vi "DepthSearch.vi"(6 "Path in":refnum<data-value>[](array[refnum]), 8 "error in (no error)":errorcluster, 10 "GraphNode in":refnum<data-value>, 11 "GraphSearch in":refnum<class "GraphSearch.lvclass">) -> (0 "error out":errorcluster, 1 "found":bool, 2 "GraphNode out":refnum<data-value>, 3 "GraphSearch out":refnum<class "GraphSearch.lvclass">, 4 "Path out":refnum<data-value>[](array[refnum]))   [LabVIEW 2009, in "GraphSearch.lvclass"]
uses:
  GraphSearch.lvclass
  GraphNode/GraphNode.lvclass
  Node/Node.lvclass
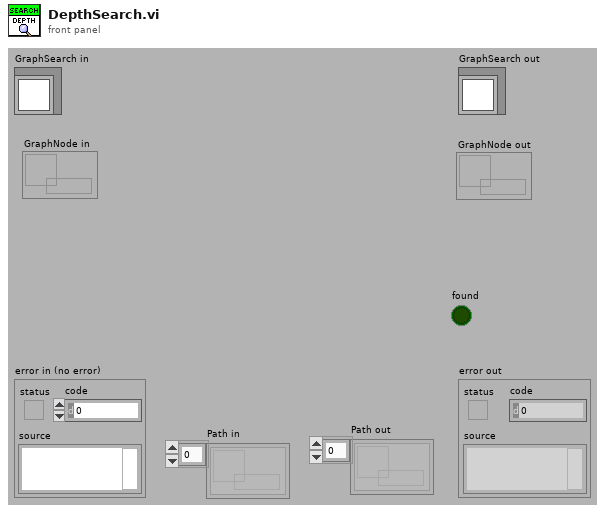
[diagram p1: front panel]
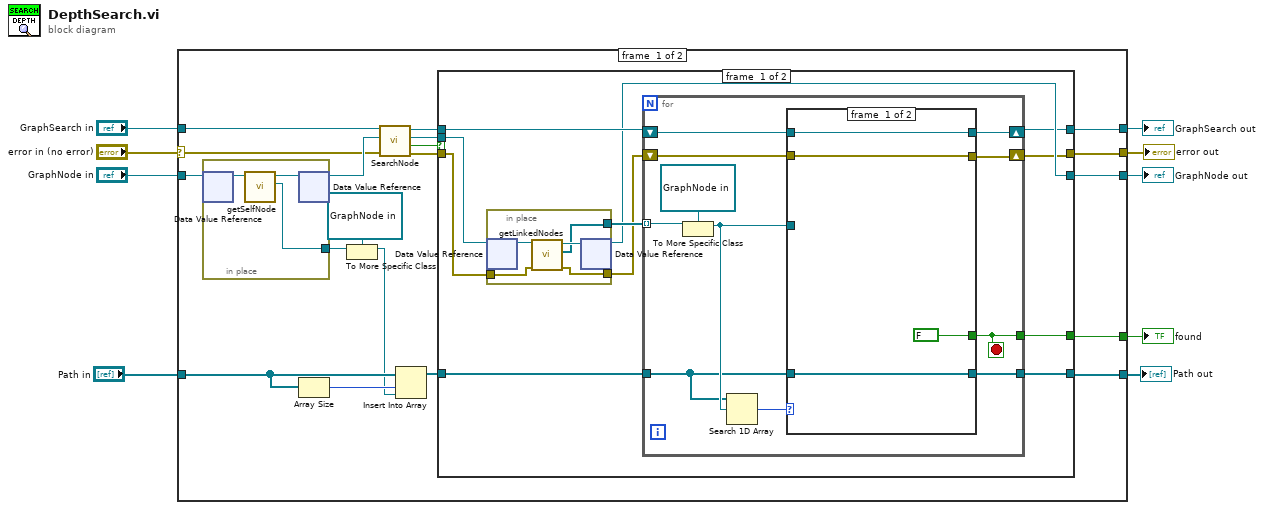
[diagram p0: block diagram]
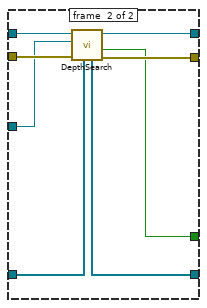
[diagram p2: hidden frame]
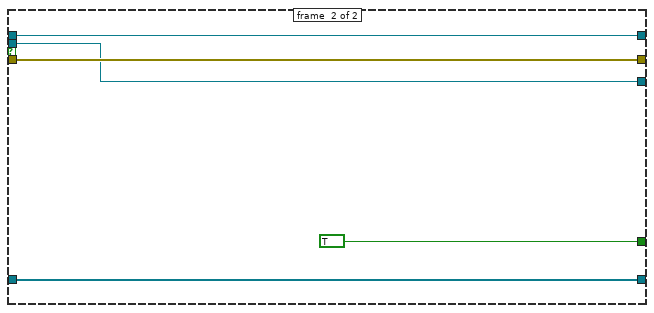
[diagram p3: hidden frame]
diagram:
  n1 = case shown="No Error" "error in (no error)" {
    selector: "error in (no error)" -> [w15 w79]
    tunnel: [w22 w79] -> w8
    tunnel: [w21 w78] -> w6
    tunnel: "GraphSearch in" -> [w19 w78]
    tunnel: "GraphNode in" -> [w18 w77]
    tunnel: "Path in" -> [w13 w76]
    tunnel: [w24 w76] -> w3
    tunnel: [w23 _] -> w2
    tunnel: [w20 w77] -> w1
    frame #0 {
      n2 = in-place {
        in-place-border: [w29] -> w16
        n3 = in-place-dvr #1(w18) -> (w31:refnum<class "GraphNode.lvclass">)  [unwired: 1 out]
        n4 = call "getSelfNode.vi"("Node in"=w31) -> ("selfNode"=w29:refnum<data-value>, "Node out"=w30:refnum<class "GraphNode.lvclass">)  [unwired: 8 in, 1 out]
        n5 = in-place-dvr #1(w30) -> (w17:refnum<data-value>)  [unwired: 1 out]
      }
      n6 = Array Size(array=w13) -> (size(s)=w11:i32)
      n7 = To More Specific Class(target class=refnum<data-value> refnum ("GraphNode out"), reference=w16) -> (specific class reference=w10:refnum<data-value>)  [unwired: 1 in, 1 out]
      n8 = call "SearchNode.vi"("error in (no error)"=w15, "GraphNode in"=w17, "GraphSearch in"=w19) -> ("error out"=w25:errorcluster, "found"=w28:bool, "GraphNode out"=w26:refnum<data-value>, "GraphSearch out"=w27:refnum<class "GraphSearch.lvclass">)  [unwired: 5 in]
      n9 = Insert Into Array(array=w13, index=w11, new element=w10) -> (w12:refnum<data-value>[])
      n10 = case shown="False" w28 {
        tunnel: w27 -> [w40 w73]
        tunnel: w26 -> [w42 w72]
        tunnel: w25 -> [w41 w74]
        tunnel: w12 -> [w38 w71]
        tunnel: [w35 w71] -> w24
        tunnel: [w37 TRUE] -> w23
        tunnel: [w33 w74] -> w22
        tunnel: [w32 w73] -> w21
        tunnel: [w34 w72] -> w20
        frame #0 {
          n11 = in-place {
            in-place-border: w41 -> [w68]
            in-place-border: [w67] -> w36
            in-place-border: [w66] -> w39
            n12 = in-place-dvr #2(w42) -> (w70:refnum<class "GraphNode.lvclass">)  [unwired: 1 out]
            n13 = call "getLinkedNodes.vi"("error in (no error)"=w68, "GraphNode in"=w70) -> ("error out"=w67:errorcluster, "LinkedNodes"=w66:refnum<data-value>[], "GraphNode out"=w69:refnum<class "GraphNode.lvclass">)  [unwired: 7 in]
            n14 = in-place-dvr #2(w69) -> (w34:refnum<data-value>)  [unwired: 1 out]
          }
          n15 = for {
            shift-right: [w52] -> w32
            shift-left: w40 -> [w53]
            tunnel: w39 -> [w51] mode=indexing
            tunnel: w38 -> [w46]
            tunnel: [w47] -> w37
            shift-right: [w44] -> w33
            shift-left: w36 -> [w45]
            tunnel: [w43] -> w35
            stop <- w47 stop-if-true
            n16 = To More Specific Class(target class=refnum<data-value> refnum ("GraphNode out"), reference=w51) -> (specific class reference=w48:refnum<data-value>)  [unwired: 1 in, 1 out]
            n17 = Search 1D Array(1D array=w46, element=w48) -> (index of element=w49:i32)  [unwired: 1 in]
            n18 = case shown="-1" w49 {
              tunnel: w53 -> [w57 w65]
              tunnel: [w57 w64] -> w52
              tunnel: w48 -> [_ w61]
              tunnel: [FALSE w60] -> w47
              tunnel: w46 -> [w54 w58]
              tunnel: w45 -> [w55 w63]
              tunnel: [w55 w62] -> w44
              tunnel: [w54 w59] -> w43
              frame #0 {
              }
              frame #1 {
                n19 = call "DepthSearch.vi"("Path in"=w58, "error in (no error)"=w63, "GraphNode in"=w61, "GraphSearch in"=w65) -> ("error out"=w62:errorcluster, "found"=w60:bool, "GraphSearch out"=w64:refnum<class "GraphSearch.lvclass">, "Path out"=w59:refnum<data-value>[])  [unwired: 3 in, 1 out]
              }
            }
          }
        }
        frame #1 {
        }
      }
    }
    frame #1 {
    }
  }
  "error out" <- w8
  "GraphSearch out" <- w6
  "Path out" <- w3
  "GraphNode out" <- w1
  "found" <- w2
